vi "buffersize.vi"(10 "Device Name":refnum<k15>="RIO0", 11 "coerced IQ rate":dbl) -> (3 "buffer size":i64)   [LabVIEW 2021]
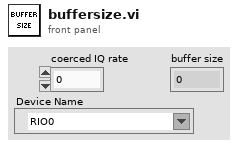
[diagram p1: front panel]
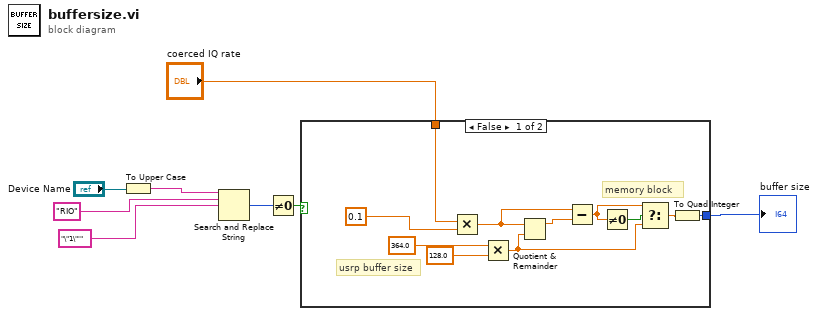
[diagram p0: block diagram]
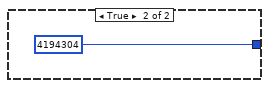
[diagram p2: hidden frame]
diagram:
  n1 = To Upper Case(1:"Device Name") -> (0:w5:string)
  n2 = Search and Replace String(input string=w5, search string="RIO", replace string="\"1\"'" ("replace string (\"\")")) -> (number of replacements=w1:i32)  [unwired: 5 in, 3 out]
  n3 = Not Equal To 0?(x=w1) -> (x != 0?=w2:bool)
  n4 = case shown="False" w2 {
    tunnel: [w19 4194304] -> w8
    tunnel: "coerced IQ rate" -> [w9 _]
    frame False {
      # "usrp buffer size"
      # "memory block"
      n5 = Multiply(x=w9, y=0.1) -> (x*y=w11:dbl)
      n6 = Multiply(x=364.0 ("y"), y=128.0) -> (x*y=w17:dbl)
      n7 = Quotient & Remainder(x=w11, y=w17) -> (x-y*floor(x/y)=w12:dbl)  [unwired: 1 out]
      n8 = Subtract(x=w11, y=w12) -> (x-y=w16:dbl)
      n9 = Not Equal To 0?(x=w16) -> (x != 0?=w15:bool)
      n10 = Select(t=w16, s=w15, f=w17) -> (s? t:f=w18:dbl)
      n11 = To Quad Integer(1:w18) -> (0:w19:i64)
    }
    frame True {
    }
  }
  "buffer size" <- w8
